vi "IPC-Core-ErrorHandlingModule.vi"(8 "error in":errorcluster, 11 "ErrorQRef":refnum<queue>) -> (0 "error out":errorcluster)   [LabVIEW 2014]
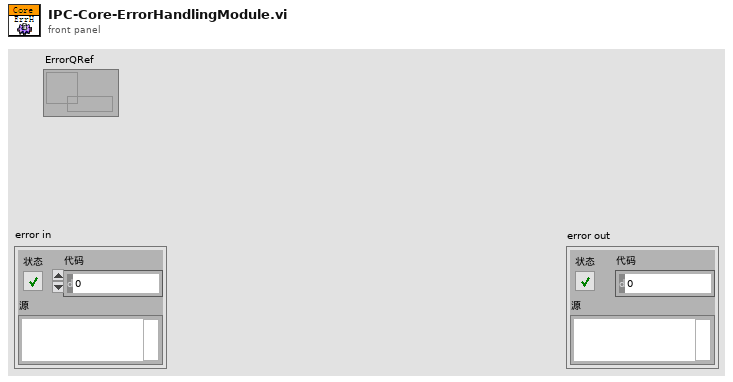
[diagram p1: front panel]
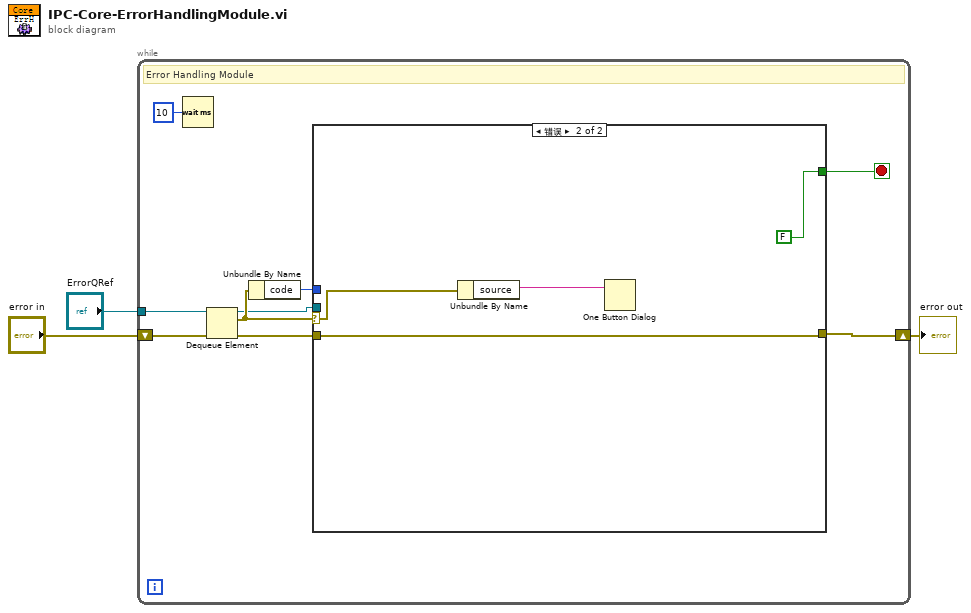
[diagram p0: block diagram]
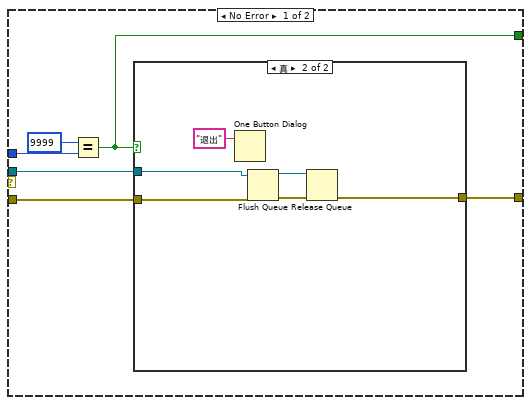
[diagram p2: hidden frame]
diagram:
  n1 = while {
    tunnel: "ErrorQRef" -> [w12]
    shift-right: [w6] -> w1
    shift-left: "error in" -> [w11]
    stop <- w7 stop-if-true
    # "Error Handling Module"
    n2 = Wait (ms)(milliseconds to wait=u32 10 ("等待时间（毫秒）")) -> ()  [unwired: 1 out]
    n3 = Dequeue Element(queue=w12, error in (no error)=w11) -> (queue out=w4:refnum<queue>, element=w9:errorcluster, error out=w5:errorcluster)  [unwired: 1 in, 1 out]
    n4 = Unbundle By Name(w9) -> ("code"=w8:i32)
    n5 = case shown="错误" w9 {
      selector: w9 -> [_ w27]
      tunnel: w8 -> [w18 _]
      tunnel: [w16 FALSE] -> w7
      tunnel: [w15 w29] -> w6
      tunnel: w5 -> [w14 w29]
      tunnel: w4 -> [w13 _]
      frame No Error {
        n6 = Equal?(x=9999, y=w18) -> (x = y?=w16:bool)
        n7 = case shown="真" w16 {
          tunnel: [w19 w23] -> w15
          tunnel: w14 -> [w19 w22]
          tunnel: w13 -> [_ w21]
          frame False {
          }
          frame True {
            n8 = One Button Dialog(message="退出" ("消息")) -> ()  [unwired: 1 in, 1 out]
            n9 = Flush Queue(queue=w21, error in (no error)=w22) -> (queue out=w25:refnum<queue>, error out=w24:errorcluster)  [unwired: 1 out]
            n10 = Release Queue(queue=w25, error in (no error)=w24) -> (error out=w23:errorcluster)  [unwired: 1 in, 2 out]
          }
        }
      }
      frame Error {
        n11 = Unbundle By Name(w27) -> ("source"=w26:string)
        n12 = One Button Dialog(message=w26) -> ()  [unwired: 1 in, 1 out]
      }
    }
  }
  "error out" <- w1
